vi "获取合法面板.vi"(11 "节点引用数组":refnum<vi>[](array[refnum])) -> (2 "数组":T1(array[cluster]), 3 "合法":bool)   [LabVIEW 2019]
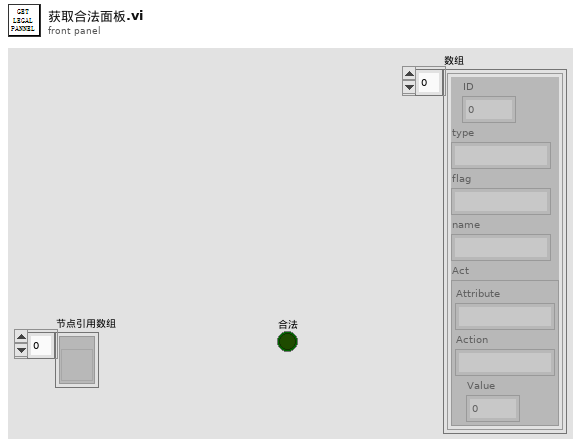
[diagram p1: front panel]
types:
  T1 = cluster{"ID":u8, "type":string, "flag":string, "name":string, "Act":cluster{"Attribute":string, "Action":string, "Value":dbl}}[]
  T2 = cluster{"ID":u8, "type":string, "flag":string, "name":string, "Act":cluster{"Attribute":string, "Action":string, "Value":dbl}}
  T3 = cluster{"Attribute":string, "Action":string, "Value":dbl}
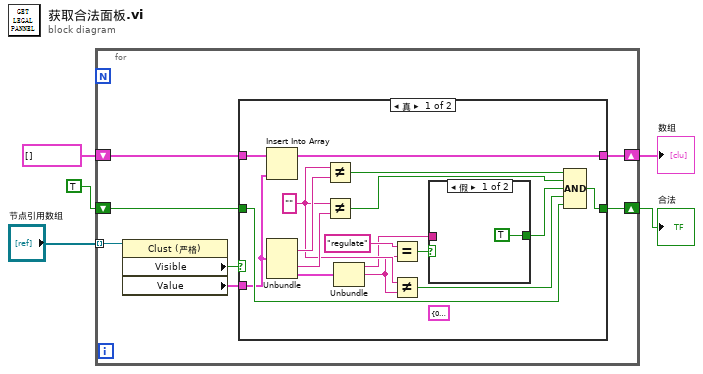
[diagram p0: block diagram]
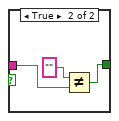
[diagram p2: hidden frame]
diagram:
  n1 = for {
    tunnel: "节点引用数组" -> [w12] mode=indexing
    shift-right: [w11] -> w3
    shift-left: TRUE -> [w10]
    shift-right: [w9] -> w2
    shift-left: T1 [] -> [w8]
    n2 = property class="Clust (严格)"(reference=w12) -> ("Visible"=w7:bool, "Value"=w6:T2)  [unwired: 1 in, 2 out]
    n3 = case shown="真" w7 {
      tunnel: [w22 w35] -> w11
      tunnel: w10 -> [w21 w35]
      tunnel: [w20 w34] -> w9
      tunnel: w8 -> [w19 w34]
      tunnel: w6 -> [w13 _]
      frame True {
        w25 = "" ("y")
        (unwired) T2 {"ID"=0, "type"="", "flag"="", "name"="", "Act"={"Attribute"="", "Action"="", "Value"=0.0}} ("Value")
        n4 = Insert Into Array(array=w19, new element=w13) -> (w20:T1)  [unwired: 1 in]
        n5 = Unbundle(w13) -> ("type"=w26:string, "name"=w27:string, "Act"=w29:T3)  [unwired: 2 out]
        n6 = Not Equal?(x=w25, y=w26) -> (x != y?=w24:bool)
        n7 = Not Equal?(x=w25, y=w27) -> (x != y?=w23:bool)
        n8 = Unbundle(w29) -> ("Attribute"=w15:string, "Action"=w17:string)  [unwired: 1 out]
        n9 = Equal?(x="regulate" ("Action"), y=w17) -> (x = y?=w16:bool)
        n10 = Not Equal?(x=w25, y=w17) -> (x != y?=w28:bool)
        n11 = case shown="假" w16 {
          tunnel: w15 -> [_ w33]
          tunnel: [TRUE w31] -> w14
          frame False {
          }
          frame True {
            n12 = Not Equal?(x="" ("y"), y=w33) -> (x != y?=w31:bool)
          }
        }
        n13 = Compound Arithmetic op=AND ("复合运算")(w24, w23, w14, w28, w21) -> (w22:bool)
      }
      frame False {
      }
    }
  }
  "合法" <- w3
  "数组" <- w2
